vi "stepExample.vi"() -> ()   [LabVIEW 2018]
uses:
  <vilib>/Instr/_visa.llb/VISA Configure Serial Port (Instr).vi
panel:
  out "error out":errorcluster
  out "read buffer":string
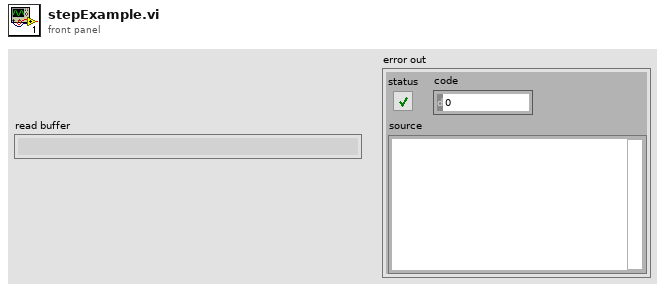
[diagram p1: front panel]
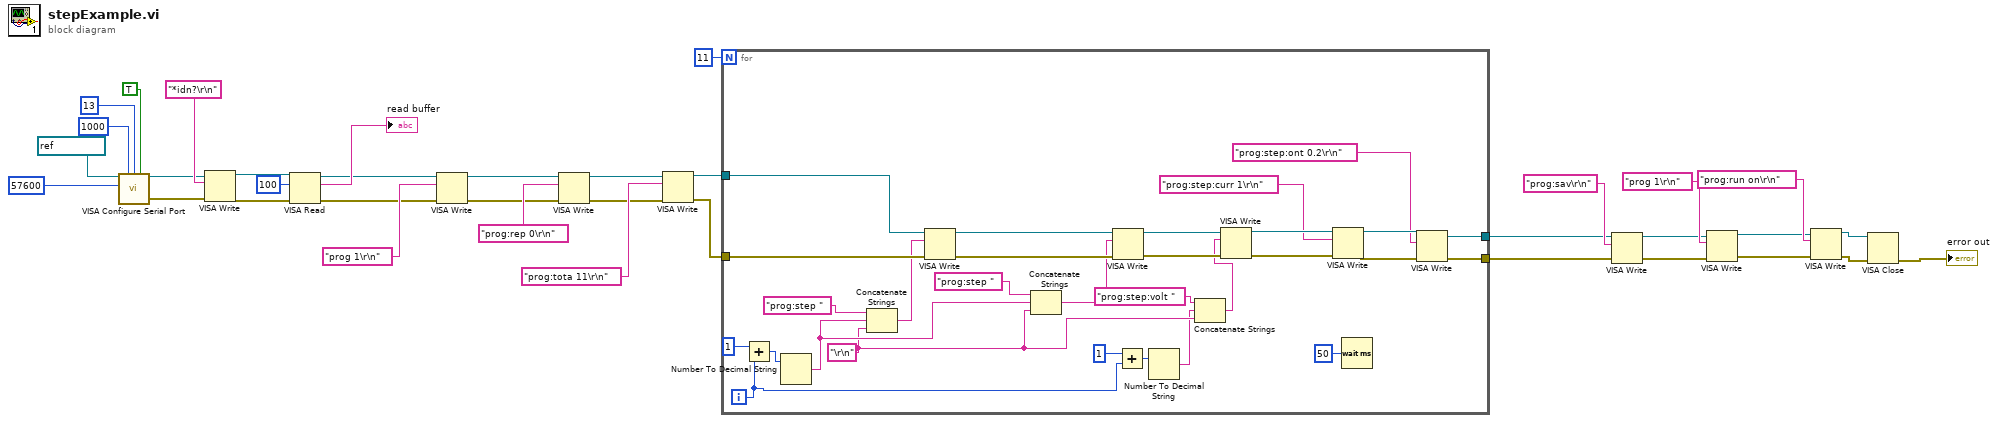
[diagram p0: block diagram]
diagram:
  n1 = call-poly "VISA Configure Serial Port"("VISA resource name"=refnum<visa-resource-name> "COM27", "timeout (10sec)"=u32 1000, "termination char\n(0xA = '\\n' = LF)"=u8 13 ("termination char\n(0xA = '\\n' = LF)"), "Enable Termination\nChar (T)"=TRUE ("Enable Termination\nChar (T)"), "baud rate (9600)"=u32 57600) -> ("VISA resource name out"=w14:refnum<visa-resource-name>, "error out"=w13:errorcluster)  [unwired: 9 in]
  n2 = VISA Write(VISA resource name=w14, write buffer="*idn?\r\n", error in (no error)=w13) -> (VISA resource name out=w33:refnum<visa-resource-name>, error out=w32:errorcluster)  [unwired: 1 out]
  n3 = VISA Read(VISA resource name=w33, byte count=u32 100, error in (no error)=w32) -> (VISA resource name out=w2:refnum<visa-resource-name>, read buffer=→"read buffer":string, error out=w1:errorcluster)  [unwired: 1 out]
  n4 = VISA Write(VISA resource name=w2, write buffer="prog 1\r\n" ("string"), error in (no error)=w1) -> (VISA resource name out=w12:refnum<visa-resource-name>, error out=w11:errorcluster)  [unwired: 1 out]
  n5 = VISA Write(VISA resource name=w12, write buffer="prog:rep 0\r\n" ("string"), error in (no error)=w11) -> (VISA resource name out=w16:refnum<visa-resource-name>, error out=w17:errorcluster)  [unwired: 1 out]
  n6 = VISA Write(VISA resource name=w16, write buffer="prog:tota 11\r\n" ("string"), error in (no error)=w17) -> (VISA resource name out=w25:refnum<visa-resource-name>, error out=w24:errorcluster)  [unwired: 1 out]
  n7 = for {
    N: 11 -> [_]
    tunnel: w25 -> [w65]
    tunnel: w24 -> [w64]
    tunnel: [w45] -> w21
    tunnel: [w44] -> w19
    i -> [w39]
    w50 = "\r\n" ("string")
    n8 = Add(x=1, y=w39) -> (x+y=w40:i32)
    n9 = Number To Decimal String(number=w40) -> (decimal integer string=w52:string)  [unwired: 1 in]
    n10 = Concatenate Strings("prog:step " ("string"), w52, w50) -> (w63:string)
    n11 = VISA Write(VISA resource name=w65, write buffer=w63, error in (no error)=w64) -> (VISA resource name out=w61:refnum<visa-resource-name>, error out=w60:errorcluster)  [unwired: 1 out]
    n12 = Concatenate Strings("prog:step " ("string"), w52, w50) -> (w54:string)
    n13 = VISA Write(VISA resource name=w61, write buffer=w54, error in (no error)=w60) -> (VISA resource name out=w59:refnum<visa-resource-name>, error out=w58:errorcluster)  [unwired: 1 out]
    n14 = Add(x=1, y=w39) -> (x+y=w42:i32)
    n15 = Number To Decimal String(number=w42) -> (decimal integer string=w41:string)  [unwired: 1 in]
    n16 = Concatenate Strings("prog:step:volt " ("string"), w41, w50) -> (w51:string)
    n17 = VISA Write(VISA resource name=w59, write buffer=w51, error in (no error)=w58) -> (VISA resource name out=w57:refnum<visa-resource-name>, error out=w56:errorcluster)  [unwired: 1 out]
    n18 = VISA Write(VISA resource name=w57, write buffer="prog:step:curr 1\r\n", error in (no error)=w56) -> (VISA resource name out=w49:refnum<visa-resource-name>, error out=w48:errorcluster)  [unwired: 1 out]
    n19 = Wait (ms)(milliseconds to wait=u32 50) -> ()  [unwired: 1 out]
    n20 = VISA Write(VISA resource name=w49, write buffer="prog:step:ont 0.2\r\n", error in (no error)=w48) -> (VISA resource name out=w44:refnum<visa-resource-name>, error out=w45:errorcluster)  [unwired: 1 out]
  }
  n21 = VISA Write(VISA resource name=w19, write buffer="prog:sav\r\n" ("string"), error in (no error)=w21) -> (VISA resource name out=w8:refnum<visa-resource-name>, error out=w7:errorcluster)  [unwired: 1 out]
  n22 = VISA Write(VISA resource name=w8, write buffer="prog 1\r\n" ("string"), error in (no error)=w7) -> (VISA resource name out=w6:refnum<visa-resource-name>, error out=w5:errorcluster)  [unwired: 1 out]
  n23 = VISA Write(VISA resource name=w6, write buffer="prog:run on\r\n" ("string"), error in (no error)=w5) -> (VISA resource name out=w4:refnum<visa-resource-name>, error out=w3:errorcluster)  [unwired: 1 out]
  n24 = VISA Close(VISA resource name=w4, error in (no error)=w3) -> (error out=→"error out":errorcluster)
